vi "Stacked Shift Register (Sum of n Numbers).vi"() -> ()   [LabVIEW 2016]
panel:
  out "Numeric 4":i32
  out "Numeric 1":i32
  out "Numeric 2":i32
  out "Numeric 3":i32
  out "Sum":i32
  in  "Input":i32
  out "Output":i32
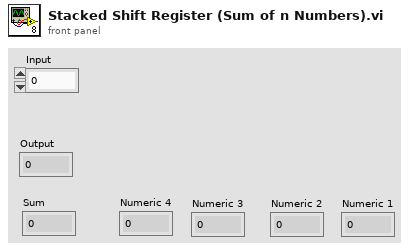
[diagram p1: front panel]
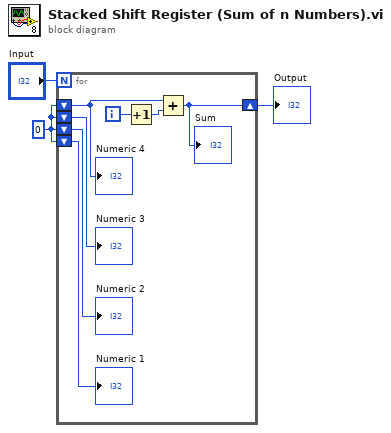
[diagram p0: block diagram]
diagram:
  w1 = 0
  n1 = for {
    N: "Input" -> [_]
    shift-right: [w8] -> w3
    shift-left: w1 -> [w4]
    shift-left: w1 -> [w7]
    shift-left: w1 -> [w6]
    shift-left: w1 -> [w5]
    i -> [w10]
    n2 = Increment(x=w10) -> (x+1=w9:i32)
    n3 = Add(x=w4, y=w9) -> (x+y=w8:i32)
    "Sum" <- w8
    "Numeric 3" <- w7
    "Numeric 2" <- w6
    "Numeric 1" <- w5
    "Numeric 4" <- w4
  }
  "Output" <- w3
